vi "Global Coude.vi"() -> ()   [LabVIEW 2018]
panel:
  out "SERIAL":T1
  out "LAMPADA":T1
  out "REDE":T1
  out "ESPELHO":T2
  out "PRISMA":T2
  out "FENDA":T2
  # "COUDE"
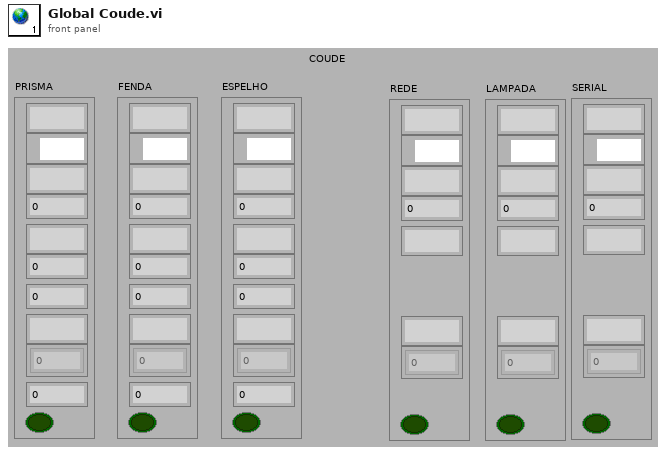
[diagram p1: front panel]
types:
  T1 = cluster{"Mec ID":string, "VISA Mec":refnum<visa-resource-name>, "Mec PosLimit":string, "Mec NegLimit":string, "MecOffset":string, "MecTargets":dbl[], "MecEnabled":bool, "Mec Target":dbl}
  T2 = cluster{"Mec ID":string, "VISA Mec":refnum<visa-resource-name>, "Mec PosLimit":string, "Mec NegLimit":string, "Mec Factor":dbl, "Mec Speed":dbl, "Mec Acceleration":dbl, "MecOffset":string, "MecTargets":dbl[], "MecEnabled":bool, "Mec Target":dbl}
diagram:
